vi "p(v).vi"(2 "v":dbl, 3 "Z":dbl, 4 "E":dbl) -> (0 "i":dbl, 1 "p":dbl)   [LabVIEW 2021]
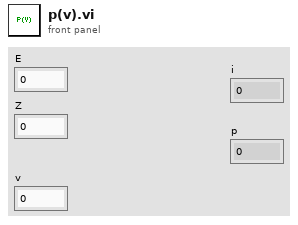
[diagram p1: front panel]
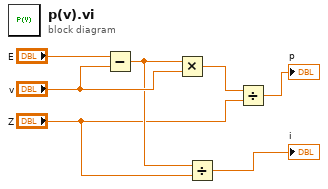
[diagram p0: block diagram]
diagram:
  n1 = Subtract(x="E", y="v") -> (x-y=w3:dbl)
  n2 = Multiply(x=w3, y="v") -> (x*y=w6:dbl)
  n3 = Divide(x=w3, y="Z") -> (x/y=→"i":dbl)
  n4 = Divide(x=w6, y="Z") -> (x/y=→"p":dbl)
